vi "Drive_StopDrive.vi"(2 "error in":errorcluster) -> (0 "error out":errorcluster)   [LabVIEW 2009, in "Drive.lvlib"]
uses:
  Drive.lvlib
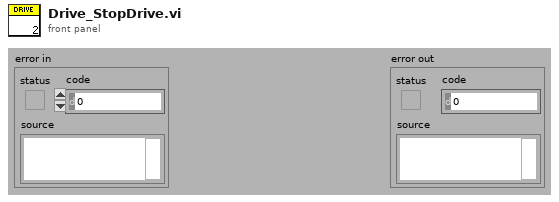
[diagram p1: front panel]
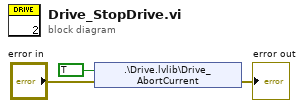
[diagram p0: block diagram]
diagram:
  n1 = shared-variable ".\\Drive.lvlib\\Drive_AbortCurrent"(TRUE ("Drive_AbortCurrent"), error in="error in") -> (error out=→"error out":errorcluster)
